vi "Update Object by Type.vi"(7 "Overwrite? (F)":bool, 8 "error in (no error)":errorcluster, 10 "Object":refnum<class>, 11 "Values in":refnum<class "Values.lvclass">) -> (0 "error out":errorcluster, 3 "Values out":refnum<class "Values.lvclass">)   [LabVIEW 2020, in "HTTP Server.lvlib" / "Values.lvclass"]
uses:
  Values.lvclass
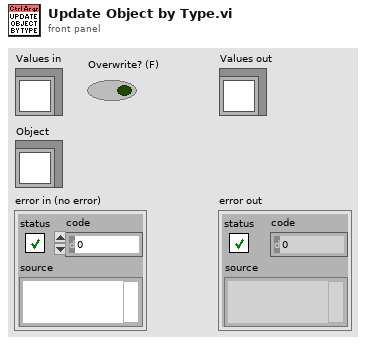
[diagram p1: front panel]
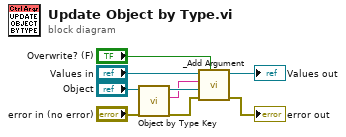
[diagram p0: block diagram]
diagram:
  n1 = call "Object by Type Key.vi"("Object In"="Object") -> ("Object Type Key"=w2:string, "Object"=w3:refnum<class>)  [unwired: 9 in]
  n2 = call "_Add Argument.vi"("Overwrite? (F)"="Overwrite? (F)", "error in (no error)"="error in (no error)", "Value"=w3, "Name"=w2, "Arguments in"="Values in") -> ("error out"=→"error out":errorcluster, "Arguments out"=→"Values out":refnum<class "Values.lvclass">)  [unwired: 5 in]
